vi "Cleanup.vi"(8 "error in (no error)":errorcluster, 11 "Mux in":refnum<class "Mux.lvclass">) -> (0 "error out":errorcluster)   [LabVIEW 2022 SP3, in "VideoMux.lvlib" / "Mux.lvclass"]
uses:
  Mux.lvclass
  Mux.lvclass/Mux.ctl
  <vilib>/IlluminatedG/lv-stream/Connection/Connection.lvclass
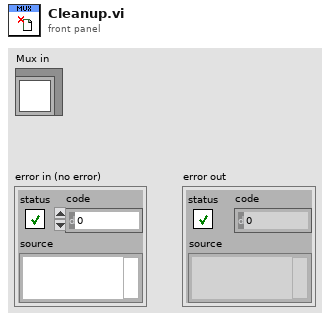
[diagram p1: front panel]
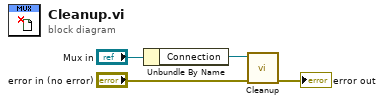
[diagram p0: block diagram]
diagram:
  n1 = Unbundle By Name("Mux in") -> ("Connection"=w3:refnum<class "Connection.lvclass">)
  n2 = call-dynamic "Cleanup.vi"("error in (no error)"="error in (no error)", "Connection in"=w3) -> ("error out"=→"error out":errorcluster)  [unwired: 9 in]
